vi "SetCreationTime.vi"(8 "error in":errorcluster, 10 "ScrappedTime":timestamp, 11 "ProductUnit in":refnum<class "ProductUnit.lvclass">) -> (0 "error out":errorcluster, 3 "ProductUnit out":refnum<class "ProductUnit.lvclass">)   [LabVIEW 2021, in "ProligentXMLGenerator.lvlib" / "ProductUnit.lvclass"]
doc: "Creation date and time of the product unit.\n\nThis attribute can't be updated after having been provided once.\n\nThis value is restricted to \"1900-01-01T00:00:00Z\" -\"2100-01-01T00:00:00Z\"."
uses:
  ProductUnit.lvclass
  ProductUnit.lvclass/ProductUnit.ctl
  Base/DateTime/DateTime.lvclass
  Base/Attribute/Attribute.lvclass
  C:/Projects/proligent-xml-generator-labview/src/ProligentXMLGenerator/Base/Attribute/Attribute.lvclass
  C:/Projects/proligent-xml-generator-labview/src/ProligentXMLGenerator/Base/DateTime/DateTime.lvclass
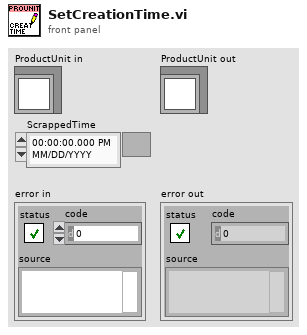
[diagram p1: front panel]
types:
  T1 = typedef "ProligentXMLGenerator.lvlib/ProductUnit.lvclass/Data.ctl" = cluster{"Name":string, "Characteristics":refnum<class "Characteristic.lvclass">[], "Documents":refnum<class "Document.lvclass">[], "CustomData":refnum<class "CustomData.lvclass">, "ProductUnitIdentifier":refnum<class "NonEmptyString_50.lvclass">, "ProductFullName":refnum<class "FullName.lvclass">, "Scrapped":refnum<class "Boolean.lvclass">, "ScrappedTime":refnum<class "DateTime.lvclass">, "CreationTime":refnum<class "DateTime.lvclass">, "ManufacturingTime":refnum<class "DateTime.lvclass">, "ByManufacturer":refnum<class "NonEmptyString_255.lvclass">, "TimeZoneInfoId":string}
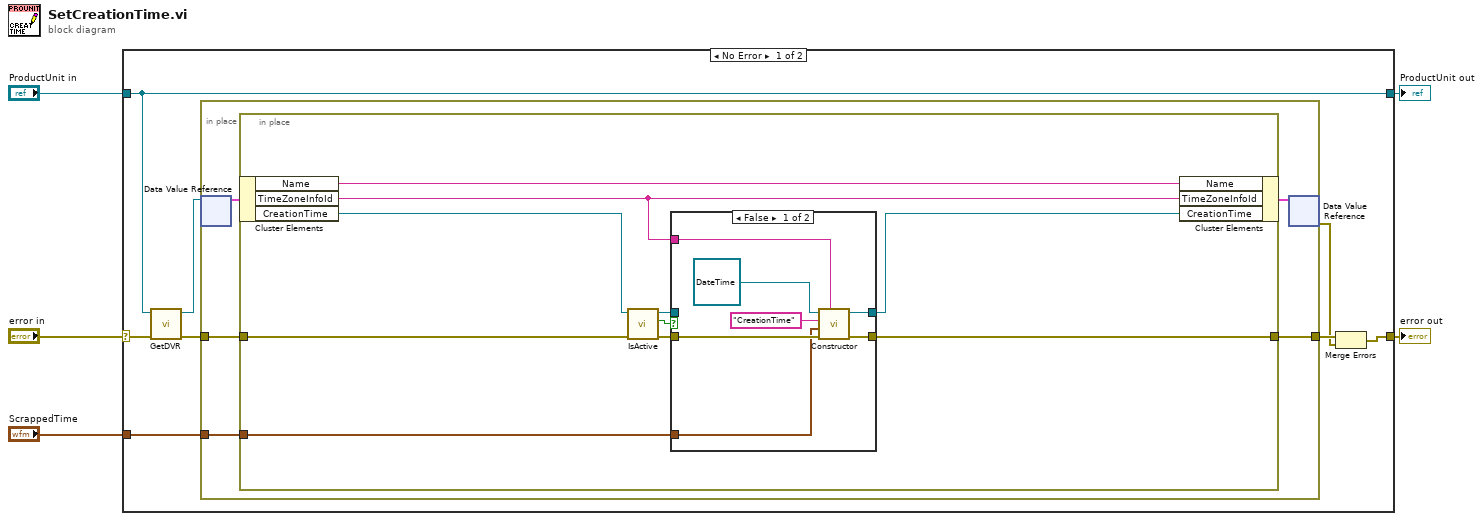
[diagram p0: block diagram]
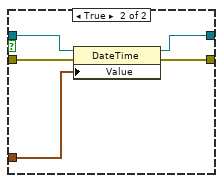
[diagram p2: hidden frame]
diagram:
  n1 = case shown="No Error" "error in" {
    selector: "error in" -> [w12 w41]
    tunnel: "ProductUnit in" -> [w7 w42]
    tunnel: [w9 w41] -> w3
    tunnel: "ScrappedTime" -> [w8 _]
    tunnel: [w7 w42] -> w1
    frame No Error {
      n2 = call "GetDVR.vi"("error in"=w12, "ProductUnit in"=w7) -> ("error out"=w11:errorcluster, "DVRReference"=w13:refnum<data-value>)  [unwired: 8 in]
      n3 = in-place "In Place Element Structure" {
        in-place-border: w11 -> [w16]
        in-place-border: [w18] -> w10
        in-place-border: w8 -> [w17]
        n4 = in-place-dvr #1(w13) -> (w15:T1)  [unwired: 1 out]
        n5 = in-place "In Place Element Structure" {
          in-place-border: [w28] -> w18
          in-place-border: w17 -> [w27]
          in-place-border: w16 -> [w23]
          n6 = in-place-cluster #2(w15) -> ("Name"=w26:string, "TimeZoneInfoId"=w19:string, "CreationTime"=w25:refnum<class "DateTime.lvclass">)
          n7 = call "IsActive.vi"("error in"=w23, "Attribute in"=w25) -> ("error out"=w22:errorcluster, "IsActive"=w20:bool, "Attribute in"=w21:refnum<class "DateTime.lvclass">)  [unwired: 7 in]
          n8 = case shown="False" w20 {
            tunnel: [w34 w40] -> w28
            tunnel: w27 -> [w31 w39]
            tunnel: w22 -> [w35 w38]
            tunnel: w21 -> [_ w37]
            tunnel: [w30 w36] -> w24
            tunnel: w19 -> [w29 _]
            frame False {
              n9 = call-dynamic "Constructor.vi"("TimeZoneInfoId"=w29, "error in"=w35, "Value"=w31, "Name"="CreationTime", "DateTime in"=refnum<class "DateTime.lvclass"> refnum ("ProligentResultProcessor:DateTime")) -> ("error out"=w34:errorcluster, "DateTime out"=w30:refnum<class "DateTime.lvclass">)  [unwired: 5 in]
            }
            frame True {
              n10 = property on="Property Node" class="DateTime"(reference=w37, error in=w38, "Value"=w39) -> (reference out=w36:refnum<class "DateTime.lvclass">, error out=w40:errorcluster)
            }
          }
          n11 = in-place-cluster #2("Name"=w26, "TimeZoneInfoId"=w19, "CreationTime"=w24) -> (w14:T1)
        }
        n12 = in-place-dvr #1(w14) -> (w6:errorcluster)  [unwired: 1 out]
      }
      n13 = Merge Errors(w10, w6) -> (w9:errorcluster)
    }
    frame Error {
    }
  }
  "error out" <- w3
  "ProductUnit out" <- w1
